vi "Create.vi"(10 "dimension size":i32, 11 "dt s":dbl) -> (3 "LinealFitting out":refnum<class "LinealFitting.lvclass">)   [LabVIEW 2019, in "LinealFitting.lvclass"]
uses:
  LinealFitting.lvclass
  LinealFitting.lvclass/LinealFitting.ctl
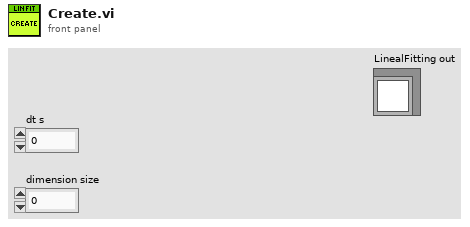
[diagram p1: front panel]
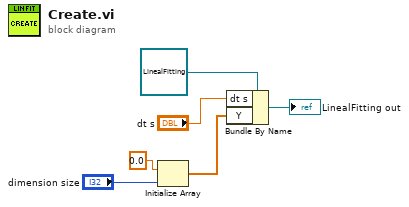
[diagram p0: block diagram]
diagram:
  n1 = Initialize Array(0.0 ("element"), "dimension size") -> (w1:dbl[])
  n2 = Bundle By Name(cluster=refnum<class "LinealFitting.lvclass"> refnum ("LinealFitting in"), "dt s"="dt s", "Y"=w1) -> (→"LinealFitting out":refnum<class "LinealFitting.lvclass">)
